vi "Modbus Multi-Write SGL.vi"(7 "Slave Address":u8, 8 "error in (no error)":errorcluster, 9 "Input data [float32]":sgl[](array[numeric]), 10 "Register Start Address":u16 format="%x", 11 "VISA resource in":refnum<visa-resource-name>) -> (0 "error out":errorcluster, 3 "VISA resource out":refnum<visa-resource-name>)   [LabVIEW 2010, in "Voegtlin_NI_SMART_Modbus_Drivers.lvlib"]
doc: "Schreibe die uebergebene Anzahl float32-Werte an die angegebene Startadresse des selektierten Geraetes.\nDer COM-Port muss dazu initialisiert sein (benutze\" Modbus Init.vi\")."
uses:
  Voegtlin_NI_SMART_Modbus_Drivers.lvlib
  Enums/Modbus Comm.ctl
panel:
  out "U16 input data to write\n(array)":u16[](array[numeric])
  # "Input Data"
  # "Internal Data"
  # "Output Data"
  # "(Inputmaske in HEX)"
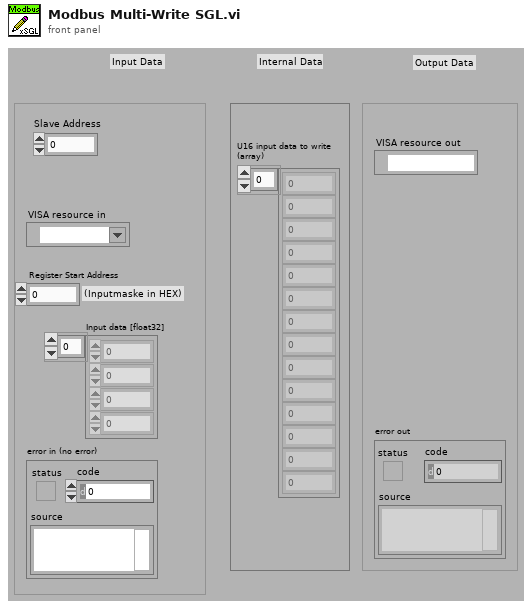
[diagram p1: front panel]
types:
  T1 = typedef "Voegtlin_NI_SMART_Modbus_Drivers.lvlib/Modbus Comm.ctl" = enum16{"Init", "Read", "Write", "Exit"}
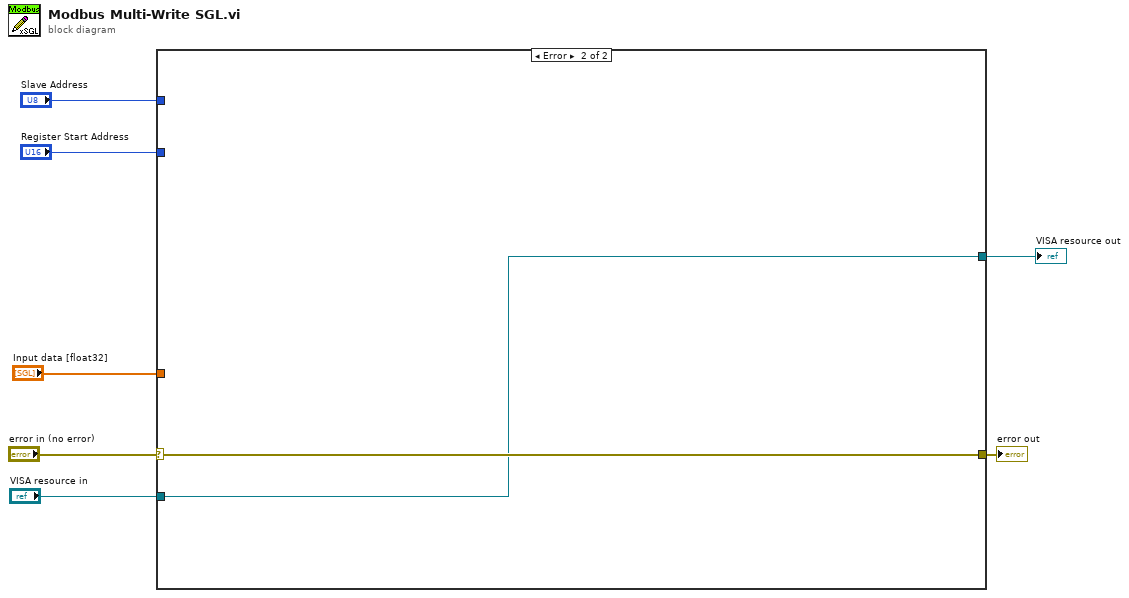
[diagram p0: block diagram]
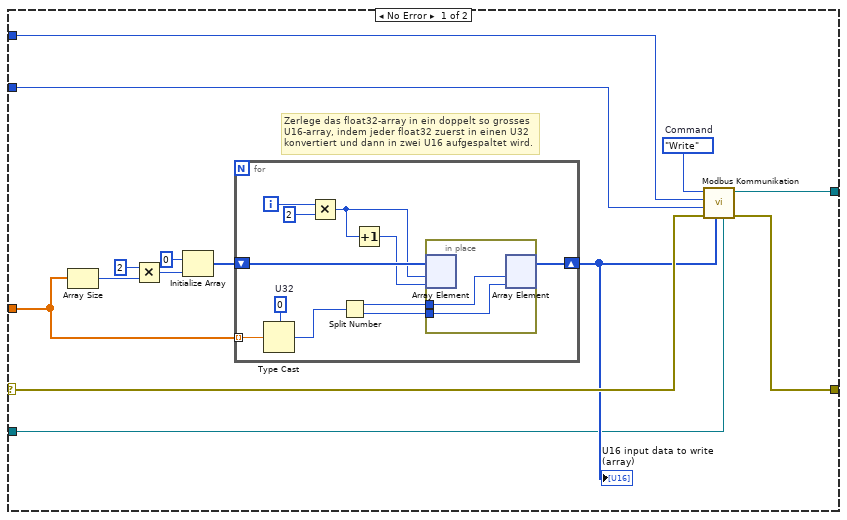
[diagram p2: hidden frame]
diagram:
  n1 = case shown="Error" "error in (no error)" {
    selector: "error in (no error)" -> [w13 w36]
    tunnel: [w20 w36] -> w7
    tunnel: "Register Start Address" -> [w11 _]
    tunnel: "Input data [float32]" -> [w14 _]
    tunnel: "Slave Address" -> [w10 _]
    tunnel: "VISA resource in" -> [w9 w35]
    tunnel: [w8 w35] -> w1
    frame No Error {
      w21 = Modbus_Comm."Write"  # Command
      # "Zerlege das float32-array in ein doppelt so grosses U16-array, indem jeder float32 zuerst in einen U32 konvertiert und dann in zwei U16 aufgespaltet wird."
      n2 = Array Size(array=w14) -> (size(s)=w19:i32)
      n3 = Multiply(x=2, y=w19) -> (x*y=w17:i32)
      n4 = Initialize Array(u16 0 ("x"), w17) -> (w15:u16[])
      n5 = for {
        shift-right: [w25] -> w12
        shift-left: w15 -> [w30]
        tunnel: w14 -> [w22] mode=indexing
        i -> [w32]
        w24 = u32 0  # U32
        n6 = Type Cast(type=w24, x=w22) -> (*(type *) &x=w23:u32)
        n7 = Multiply(x=w32, y=2) -> (x*y=w29:i32)
        n8 = Split Number(x=w23) -> (hi(x)=w27:u16, lo(x)=w26:u16)
        n9 = Increment(x=w29) -> (x+1=w28:i32)
        n10 = in-place {
          in-place-border: w27 -> [w34]
          in-place-border: w26 -> [w33]
          n11 = in-place-array #1(w30, w29, w28) -> ()  [unwired: 2 out]
          n12 = in-place-array #1(w34, w33) -> (w25:u16[])  [unwired: 2 out]
        }
      }
      "U16 input data to write\n(array)" <- w12
      n13 = call "Modbus Kommunikation.vi"("VISA resource in"=w9, "Data In / #Reads [U16]"=w12, "error in (no error)"=w13, "Register Start Address"=w11, "Slave Address"=w10, "Command"=w21) -> ("error out"=w20:errorcluster, "VISA resource out"=w8:refnum<visa-resource-name>)  [unwired: 3 in, 1 out]
    }
    frame Error {
    }
  }
  "error out" <- w7
  "VISA resource out" <- w1
